vi "分频器（I32).vi"(1 "0有效？":bool=TRUE, 2 "In":i32, 4 "n":i32=2) -> (6 "Out":bool)   [LabVIEW 2012]
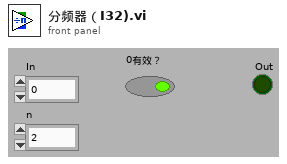
[diagram p1: front panel]
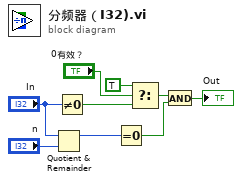
[diagram p0: block diagram]
diagram:
  n1 = Quotient & Remainder(x="In", y="n") -> (x-y*floor(x/y)=w8:i32)  [unwired: 1 out]
  n2 = Not Equal To 0?(x="In") -> (x != 0?=w4:bool)
  n3 = Equal To 0?(x=w8) -> (x = 0?=w6:bool)
  n4 = Select(t=TRUE, s="0有效？", f=w4) -> (s? t:f=w3:bool)
  n5 = And(x=w3, y=w6) -> (x .and. y?=→"Out":bool)
